vi "9402_Update Lines.vi"(8 "error in (no error)":errorcluster, 10 "Line directions":u32[](array[ring]) items=["Input", "Output"], 11 "Node Ptr in":T1 format="%.0x") -> (0 "error out":errorcluster, 3 "Node Ptr out":T1 format="%.0x")   [LabVIEW 2019, in "Modules.lvlib" / "9402.lvclass"]
uses:
  9402.lvclass
  <vilib>/NI VeriStand/Custom Device API/Custom Device Item Ref.ctl
  C:/Users/nitest/Desktop/Git 2019/niveristand-scan-engine-module-libraries/Source/RSI Module/RSI Module.lvclass
  <vilib>/NI VeriStand/Custom Device API/Custom Device Channel Type.ctl
  9402.lvclass/9402.ctl
  RSI Module/Channel GUIDs.vi
  RSI Module/RSI Module.lvclass
  <vilib>/NI VeriStand/Custom Device API/Custom Device API.lvlib
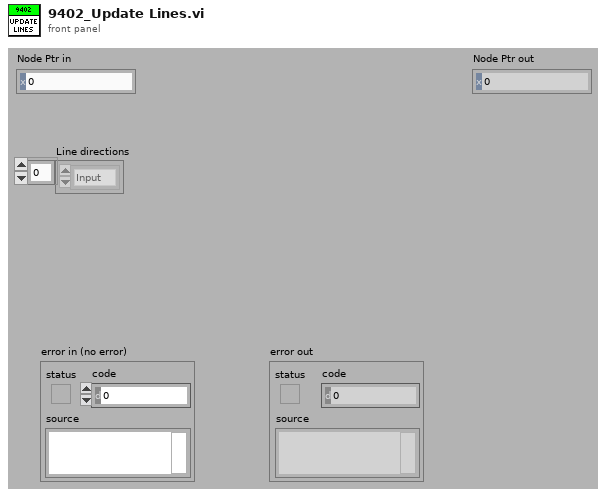
[diagram p1: front panel]
types:
  T1 = typedef "Custom Device API.lvlib/Custom Device Item Ref.ctl" = u64
  T2 = typedef "Custom Device API.lvlib/Custom Device Channel Type.ctl" = enum16{"Input", "Output"}
  T3 = typedef "Modules.lvlib/RSI Module.lvclass/Channels.ctl" = cluster{"# Input Channels":i32, "# Output Channels":i32, "Channel Type":T4, "Units":string}
  T4 = typedef "Modules.lvlib/RSI Module.lvclass/Channel Type.ctl" = enum16{"Analog", "Digital"}
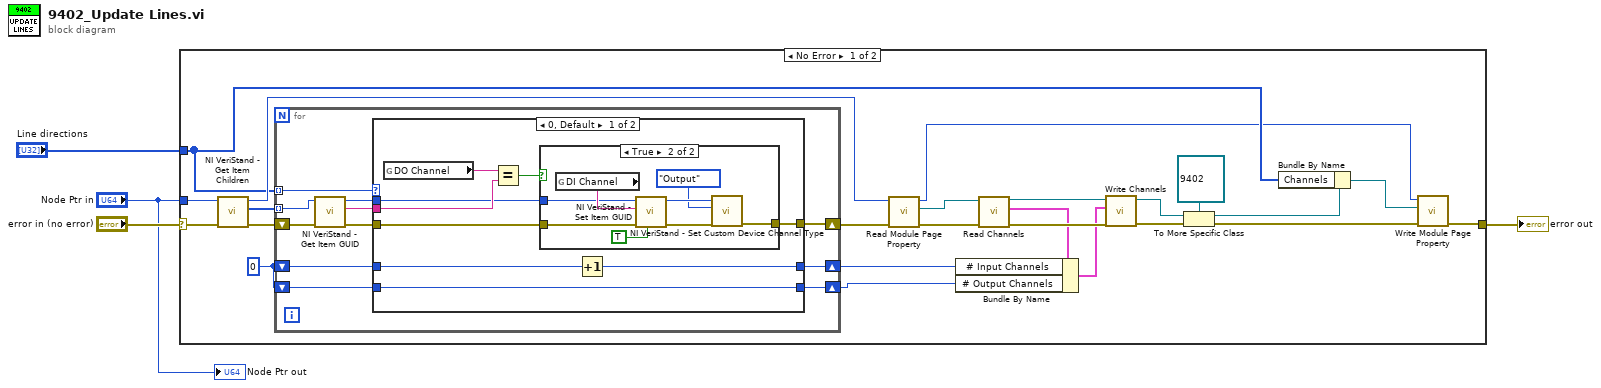
[diagram p0: block diagram]
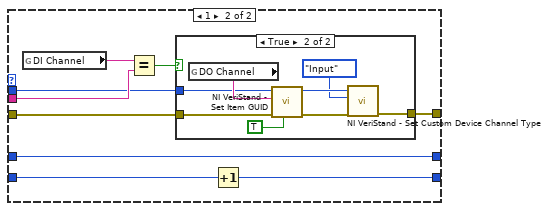
[diagram p3: hidden frame]
diagram:
  n1 = case shown="No Error" "error in (no error)" {
    selector: "error in (no error)" -> [w17 w76]
    tunnel: [w5 w76] -> w3
    tunnel: "Node Ptr in" -> [w16 _]
    tunnel: "Line directions" -> [w13 _]
    frame No Error {
      w24 = 0 ("# Input Channels")
      n2 = call <vilib>:"NI VeriStand - Get Item Children.vi"("error in (no error)"=w17, "Item Ref in"=w16) -> ("error out"=w25:errorcluster, "Child Refs"=w26:T1[], "Item Ref out"=w14:T1)  [unwired: 6 in, 1 out]
      n3 = for {
        tunnel: w26 -> [w38] mode=indexing
        tunnel: w13 -> [w37] mode=indexing
        shift-right: [w33] -> w15
        shift-left: w25 -> [w39]
        shift-right: [w30] -> w20
        shift-left: w24 -> [w32]
        shift-right: [w29] -> w19
        shift-left: w24 -> [w31]
        n4 = call <vilib>:"NI VeriStand - Get Item GUID.vi"("error in (no error)"=w39, "Item Ref in"=w38) -> ("error out"=w34:errorcluster, "GUID"=w36:string, "Item Ref out"=w35:T1)  [unwired: 7 in]
        n5 = case shown="0, Default" w37 {
          tunnel: w36 -> [w47 w65]
          tunnel: w35 -> [w44 w62]
          tunnel: w34 -> [w45 w63]
          tunnel: [w43 w61] -> w33
          tunnel: w32 -> [w42 w58]
          tunnel: w31 -> [w40 w60]
          tunnel: [w41 w58] -> w30
          tunnel: [w40 w59] -> w29
          frame 0, Default {
            n6 = global read "Channel GUIDs.vi" "DO Channel"() -> (w48:string)
            n7 = Equal?(x=w48, y=w47) -> (x = y?=w46:bool)
            n8 = case shown="True" w46 {
              tunnel: w45 -> [w49 w57]
              tunnel: w44 -> [_ w55]
              tunnel: [w49 w52] -> w43
              frame False {
              }
              frame True {
                n9 = global read "Channel GUIDs.vi" "DI Channel"() -> (w56:string)
                n10 = call <vilib>:"NI VeriStand - Set Item GUID.vi"("Refresh System Explorer Tree? (F)"=TRUE, "error in (no error)"=w57, "GUID"=w56, "Item Ref in"=w55) -> ("error out"=w53:errorcluster, "Item Ref out"=w54:T1)  [unwired: 6 in]
                n11 = call <vilib>:"NI VeriStand - Set Custom Device Channel Type.vi"("error in (no error)"=w53, "Type"=Custom_Device_Channel_Type."Output", "Channel Ref in"=w54) -> ("error out"=w52:errorcluster)  [unwired: 7 in, 1 out]
              }
            }
            n12 = Increment(x=w42) -> (x+1=w41:i32)
          }
          frame 1 {
            n13 = global read "Channel GUIDs.vi" "DI Channel"() -> (w66:string)
            n14 = Equal?(x=w66, y=w65) -> (x = y?=w64:bool)
            n15 = case shown="True" w64 {
              tunnel: w63 -> [w67 w75]
              tunnel: w62 -> [_ w73]
              tunnel: [w67 w70] -> w61
              frame False {
              }
              frame True {
                n16 = global read "Channel GUIDs.vi" "DO Channel"() -> (w74:string)
                n17 = call <vilib>:"NI VeriStand - Set Item GUID.vi"("Refresh System Explorer Tree? (F)"=TRUE, "error in (no error)"=w75, "GUID"=w74, "Item Ref in"=w73) -> ("error out"=w71:errorcluster, "Item Ref out"=w72:T1)  [unwired: 6 in]
                n18 = call <vilib>:"NI VeriStand - Set Custom Device Channel Type.vi"("error in (no error)"=w71, "Type"=Custom_Device_Channel_Type."Input", "Channel Ref in"=w72) -> ("error out"=w70:errorcluster)  [unwired: 7 in, 1 out]
              }
            }
            n19 = Increment(x=w60) -> (x+1=w59:i32)
          }
        }
      }
      n20 = call "Read Module Page Property.vi"("error in (no error)"=w15, "Node Ptr In"=w14) -> ("error out"=w11:errorcluster, "RSI Module"=w12:refnum<class "RSI Module.lvclass">, "Node Ptr Out"=w6:T1)  [unwired: 7 in]
      n21 = call "Read Channels.vi"("error in (no error)"=w11, "RSI Module in"=w12) -> ("error out"=w23:errorcluster, "Channels"=w21:T3, "RSI Module out"=w22:refnum<class "RSI Module.lvclass">)  [unwired: 7 in]
      n22 = Bundle By Name(cluster=w21, "# Input Channels"=w20, "# Output Channels"=w19) -> (w18:T3)
      n23 = call "Write Channels.vi"("error in (no error)"=w23, "Channels"=w18, "RSI Module in"=w22) -> ("error out"=w9:errorcluster, "RSI Module out"=w10:refnum<class "RSI Module.lvclass">)  [unwired: 7 in]
      n24 = To More Specific Class(target class=refnum<class "9402.lvclass"> refnum ("9205 in"), reference=w10, error in=w9) -> (specific class reference=w27:refnum<class "9402.lvclass">, error out=w7:errorcluster)
      n25 = Bundle By Name(cluster=w27, "Channels"=w13) -> (w8:refnum<class "9402.lvclass">)
      n26 = call "Write Module Page Property.vi"("error in (no error)"=w7, "RSI Module"=w8, "Node Ptr In"=w6) -> ("error out"=w5:errorcluster)  [unwired: 6 in, 2 out]
    }
    frame Error {
    }
  }
  "error out" <- w3
  "Node Ptr out" <- "Node Ptr in"
